vi "Byte Buffer.Write.Typed Array.vi"(0 "Byte Buffer in":refnum<class "Byte Buffer.lvclass">, 1 "data type":T1, 5 "buffer in":dbl[](array[numeric]), 7 "count":i64, 9 "buffer offset":u64, 11 "error in (no error)":errorcluster) -> (4 "Byte Buffer out":refnum<class "Byte Buffer.lvclass">, 6 "buffer out":dbl[](array[numeric]), 10 "new buffer offset":u64, 15 "error out":errorcluster)   [LabVIEW 2016, in "VeriStand Data.lvlib" / "Byte Buffer.lvclass"]
uses:
  Byte Buffer.lvclass
  Typedefs/Typedefs.Data Types.ctl
  Byte Buffer.lvclass/Byte Buffer.ctl
  Byte Buffer.Write (1D Boolean).vi
  Type Conversion/Type Conversion.From Double.Subset (1D Boolean).vi
  Byte Buffer.Write (1D SGL).vi
  Type Conversion/Type Conversion.From Double.Subset (1D SGL).vi
  Byte Buffer.Write (1D DBL).vi
  Byte Buffer.Write (1D I8).vi
  Type Conversion/Type Conversion.From Double.Subset (1D I8).vi
  Byte Buffer.Write (1D I16).vi
  Type Conversion/Type Conversion.From Double.Subset (1D I16).vi
  Byte Buffer.Write (1D I32).vi
  Type Conversion/Type Conversion.From Double.Subset (1D I32).vi
  Byte Buffer.Write (1D I64).vi
  Type Conversion/Type Conversion.From Double.Subset (1D I64).vi
  Byte Buffer.Write (1D U8).vi
  Type Conversion/Type Conversion.From Double.Subset (1D U8).vi
  Byte Buffer.Write (1D U16).vi
  Type Conversion/Type Conversion.From Double.Subset (1D U16).vi
  Byte Buffer.Write (1D U32).vi
  Type Conversion/Type Conversion.From Double.Subset (1D U32).vi
  Byte Buffer.Write (1D U64).vi
  Type Conversion/Type Conversion.From Double.Subset (1D U64).vi
  Byte Buffer.Write (String).vi
  Type Conversion/Type Conversion.From Double.vi
  Type Conversion/Type Conversion.From Double (1D Boolean).vi
  Type Conversion/Type Conversion.From Double (1D SGL).vi
  Type Conversion/Type Conversion.From Double (1D I8).vi
  Type Conversion/Type Conversion.From Double (1D I16).vi
  Type Conversion/Type Conversion.From Double (1D I32).vi
  Type Conversion/Type Conversion.From Double (1D I64).vi
  Type Conversion/Type Conversion.From Double (1D U8).vi
  Type Conversion/Type Conversion.From Double (1D U16).vi
  Type Conversion/Type Conversion.From Double (1D U32).vi
  Type Conversion/Type Conversion.From Double (1D U64).vi
  Utilities/Utilities.Sizeof.Scalar.vi
  Byte Buffer.Buffer Subset.Set.vi
  Memory Management/Memory Management.MoveByteBlock.Read (String).vi
  Memory Management/Memory Management.Handle Return.vi
  VeriStand Data.lvlib
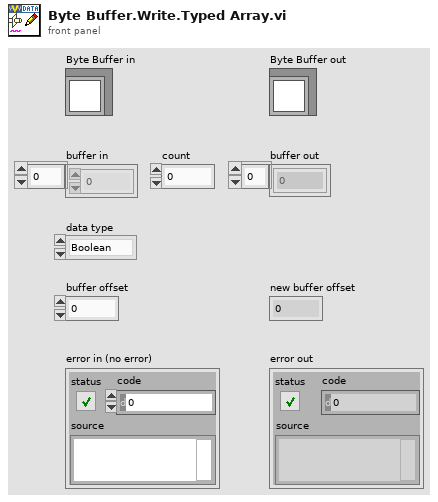
[diagram p1: front panel]
types:
  T1 = typedef "VeriStand Data.lvlib/Typedefs.Data Types.ctl" = enum16{"Boolean", "Single", "Double", "I8", "I16", "I32", "I64", "U8", "U16", "U32", "U64"}
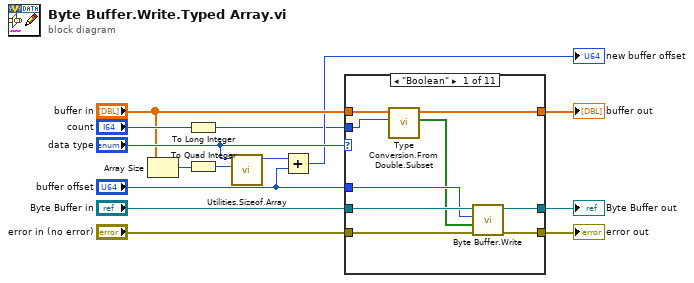
[diagram p0: block diagram]
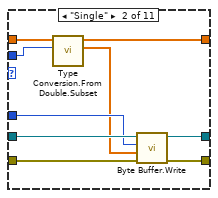
[diagram p2: hidden frame]
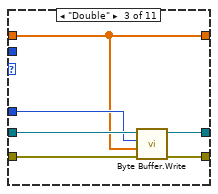
[diagram p3: hidden frame]
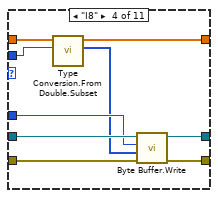
[diagram p4: hidden frame]
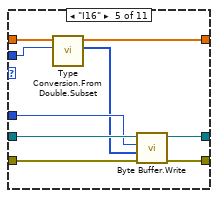
[diagram p5: hidden frame]
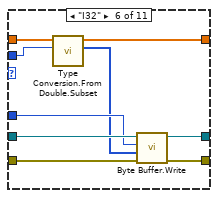
[diagram p6: hidden frame]
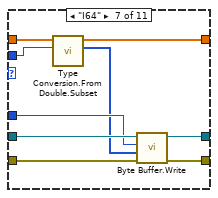
[diagram p7: hidden frame]
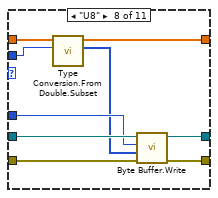
[diagram p8: hidden frame]
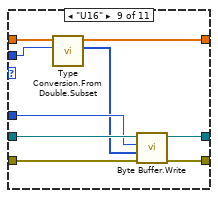
[diagram p9: hidden frame]
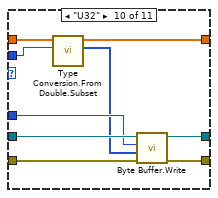
[diagram p10: hidden frame]
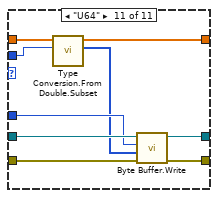
[diagram p11: hidden frame]
diagram:
  n1 = Array Size(array="buffer in") -> (size(s)=w11:i32)
  n2 = To Long Integer(number="count") -> (32bit integer=w2:i32)
  n3 = To Quad Integer(1:w11) -> (0:w1:i64)
  n4 = call "Utilities.Sizeof.Array.vi"("count"=w1, "data type"="data type") -> ("size"=w6:u64)  [unwired: 9 in]
  n5 = Add(x=w6, y="buffer offset") -> (x+y=→"new buffer offset":u64)
  n6 = case shown="\"Boolean\"" "data type" {
    tunnel: "buffer in" -> [w23 w32 w33 w47 w56 w65 w74 w83 w92 w101 w110]
    tunnel: "buffer offset" -> [w20 w29 w36 w44 w53 w62 w71 w80 w89 w98 w107]
    tunnel: "Byte Buffer in" -> [w22 w31 w38 w46 w55 w64 w73 w82 w91 w100 w109]
    tunnel: [w21 w30 w37 w45 w54 w63 w72 w81 w90 w99 w108] -> w14
    tunnel: "error in (no error)" -> [w19 w28 w35 w43 w52 w61 w70 w79 w88 w97 w106]
    tunnel: [w18 w27 w34 w42 w51 w60 w69 w78 w87 w96 w105] -> w12
    tunnel: [w17 w26 w33 w41 w50 w59 w68 w77 w86 w95 w104] -> w9
    tunnel: w2 -> [w16 w25 _ w40 w49 w58 w67 w76 w85 w94 w103]
    frame "Boolean" {
      n7 = call-poly "Type Conversion.From Double.Subset.vi"("count"=w16, "values in"=w23) -> ("converted values out"=w15:bool[], "values out"=w17:dbl[])  [unwired: 8 in]
      n8 = call-poly "Byte Buffer.Write.vi"("error in (no error)"=w19, "values"=w15, "buffer offset"=w20, "Byte Buffer in"=w22) -> ("error out"=w18:errorcluster, "Byte Buffer out"=w21:refnum<class "Byte Buffer.lvclass">)  [unwired: 6 in]
    }
    frame "Single" {
      n9 = call-poly "Type Conversion.From Double.Subset.vi"("count"=w25, "values in"=w32) -> ("converted values out"=w24:sgl[], "values out"=w26:dbl[])  [unwired: 8 in]
      n10 = call-poly "Byte Buffer.Write.vi"("error in (no error)"=w28, "values"=w24, "buffer offset"=w29, "Byte Buffer in"=w31) -> ("error out"=w27:errorcluster, "Byte Buffer out"=w30:refnum<class "Byte Buffer.lvclass">)  [unwired: 6 in]
    }
    frame "Double" {
      n11 = call-poly "Byte Buffer.Write.vi"("error in (no error)"=w35, "values"=w33, "buffer offset"=w36, "Byte Buffer in"=w38) -> ("error out"=w34:errorcluster, "Byte Buffer out"=w37:refnum<class "Byte Buffer.lvclass">)  [unwired: 6 in]
    }
    frame "I8" {
      n12 = call-poly "Type Conversion.From Double.Subset.vi"("count"=w40, "values in"=w47) -> ("converted values out"=w39:i8[], "values out"=w41:dbl[])  [unwired: 8 in]
      n13 = call-poly "Byte Buffer.Write.vi"("error in (no error)"=w43, "values"=w39, "buffer offset"=w44, "Byte Buffer in"=w46) -> ("error out"=w42:errorcluster, "Byte Buffer out"=w45:refnum<class "Byte Buffer.lvclass">)  [unwired: 6 in]
    }
    frame "I16" {
      n14 = call-poly "Type Conversion.From Double.Subset.vi"("count"=w49, "values in"=w56) -> ("converted values out"=w48:i16[], "values out"=w50:dbl[])  [unwired: 8 in]
      n15 = call-poly "Byte Buffer.Write.vi"("error in (no error)"=w52, "values"=w48, "buffer offset"=w53, "Byte Buffer in"=w55) -> ("error out"=w51:errorcluster, "Byte Buffer out"=w54:refnum<class "Byte Buffer.lvclass">)  [unwired: 6 in]
    }
    frame "I32" {
      n16 = call-poly "Type Conversion.From Double.Subset.vi"("count"=w58, "values in"=w65) -> ("converted values out"=w57:i32[], "values out"=w59:dbl[])  [unwired: 8 in]
      n17 = call-poly "Byte Buffer.Write.vi"("error in (no error)"=w61, "values"=w57, "buffer offset"=w62, "Byte Buffer in"=w64) -> ("error out"=w60:errorcluster, "Byte Buffer out"=w63:refnum<class "Byte Buffer.lvclass">)  [unwired: 6 in]
    }
    frame "I64" {
      n18 = call-poly "Type Conversion.From Double.Subset.vi"("count"=w67, "values in"=w74) -> ("converted values out"=w66:i64[], "values out"=w68:dbl[])  [unwired: 8 in]
      n19 = call-poly "Byte Buffer.Write.vi"("error in (no error)"=w70, "values"=w66, "buffer offset"=w71, "Byte Buffer in"=w73) -> ("error out"=w69:errorcluster, "Byte Buffer out"=w72:refnum<class "Byte Buffer.lvclass">)  [unwired: 6 in]
    }
    frame "U8" {
      n20 = call-poly "Type Conversion.From Double.Subset.vi"("count"=w76, "values in"=w83) -> ("converted values out"=w75:u8[], "values out"=w77:dbl[])  [unwired: 8 in]
      n21 = call-poly "Byte Buffer.Write.vi"("error in (no error)"=w79, "values"=w75, "buffer offset"=w80, "Byte Buffer in"=w82) -> ("error out"=w78:errorcluster, "Byte Buffer out"=w81:refnum<class "Byte Buffer.lvclass">)  [unwired: 6 in]
    }
    frame "U16" {
      n22 = call-poly "Type Conversion.From Double.Subset.vi"("count"=w85, "values in"=w92) -> ("converted values out"=w84:u16[], "values out"=w86:dbl[])  [unwired: 8 in]
      n23 = call-poly "Byte Buffer.Write.vi"("error in (no error)"=w88, "values"=w84, "buffer offset"=w89, "Byte Buffer in"=w91) -> ("error out"=w87:errorcluster, "Byte Buffer out"=w90:refnum<class "Byte Buffer.lvclass">)  [unwired: 6 in]
    }
    frame "U32" {
      n24 = call-poly "Type Conversion.From Double.Subset.vi"("count"=w94, "values in"=w101) -> ("converted values out"=w93:u32[], "values out"=w95:dbl[])  [unwired: 8 in]
      n25 = call-poly "Byte Buffer.Write.vi"("error in (no error)"=w97, "values"=w93, "buffer offset"=w98, "Byte Buffer in"=w100) -> ("error out"=w96:errorcluster, "Byte Buffer out"=w99:refnum<class "Byte Buffer.lvclass">)  [unwired: 6 in]
    }
    frame "U64" {
      n26 = call-poly "Type Conversion.From Double.Subset.vi"("count"=w103, "values in"=w110) -> ("converted values out"=w102:u64[], "values out"=w104:dbl[])  [unwired: 8 in]
      n27 = call-poly "Byte Buffer.Write.vi"("error in (no error)"=w106, "values"=w102, "buffer offset"=w107, "Byte Buffer in"=w109) -> ("error out"=w105:errorcluster, "Byte Buffer out"=w108:refnum<class "Byte Buffer.lvclass">)  [unwired: 6 in]
    }
  }
  "error out" <- w12
  "Byte Buffer out" <- w14
  "buffer out" <- w9
